vi "RT Write to Serial.vi"(4 "FPGA VI Reference in":refnum<k20>, 5 "FPGA version":string="N/A", 6 "RT Main version":string="N/A", 7 "error in":errorcluster, 8 "timeout in ms":i32=20, 9 "queue in":refnum<queue>, 10 "port name in":refnum<visa-resource-name>) -> (0 "error out":errorcluster, 2 "message dequeued?":bool, 3 "port name out":refnum<visa-resource-name>)   [LabVIEW 2018]
uses:
  Type Def Ctrls/RT ctrls/data summary.ctl
  <vilib>/Utility/error.llb/whitespace.ctl
  <vilib>/NI_Real-Time Target Support.lvlib
panel:
  out "concatenated string":string
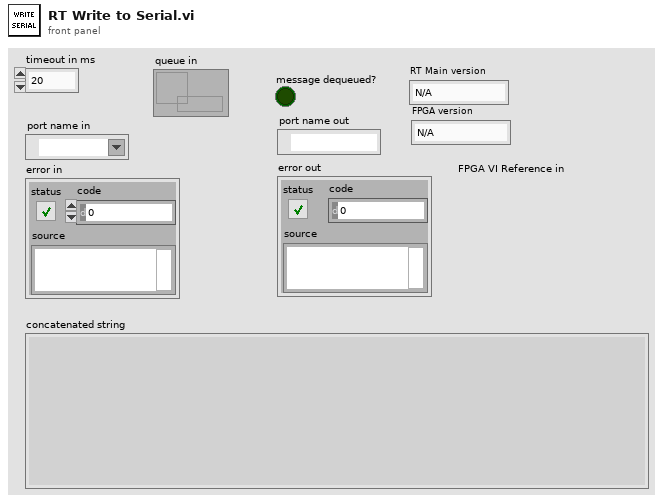
[diagram p1: front panel]
types:
  T1 = typedef "data summary.ctl" = cluster{"TIMESTAMP":dbl, "INPUT_CHN_DATA":sgl[], "OUTPUT_CHN_DATA":sgl[], "CJC_TEMPERATURE":sgl, "RELAY_SETTING":u32, "REQUEST_ID":u64, "update_system_status?":bool, "update_error_log?":bool}
  T2 = cluster{"0. connect/reconnect?":bool, "last: disconnect?":bool, "slow serial port init delay":u32}
  T3 = cluster{"2: expecting response?":bool, "expected max length":u32}
  T4 = cluster{"1: do writing?":bool, "write buffer":string}
  T5 = typedef "whitespace.ctl" = u16
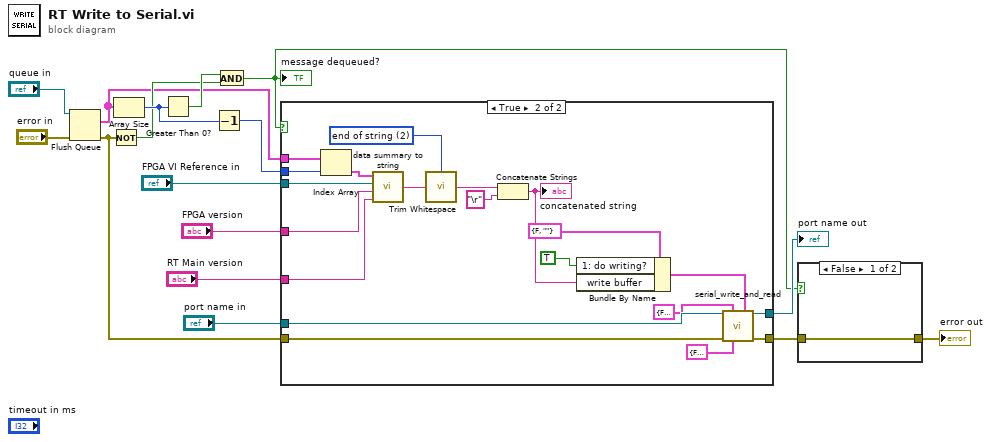
[diagram p0: block diagram]
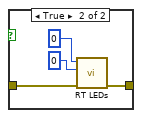
[diagram p2: hidden frame]
diagram:
  n1 = Flush Queue(queue="queue in", error in (no error)="error in") -> (remaining elements=w2:T1[], error out=w10:errorcluster)  [unwired: 1 out]
  n2 = Not(x=w10) -> (.not. x?=w7:bool)
  n3 = Array Size(array=w2) -> (size(s)=w9:i32)
  n4 = Greater Than 0?(x=w9) -> (x > 0?=w8:bool)
  n5 = Decrement(x=w9) -> (x-1=w1:i32)
  n6 = And(x=w8, y=w7) -> (x .and. y?=w6:bool)
  "message dequeued?" <- w6
  n7 = case shown="True" w6 {
    tunnel: "port name in" -> [w17 w38]
    tunnel: w10 -> [w18 w37]
    tunnel: [w18 w36] -> w14
    tunnel: [w17 w35] -> w13
    tunnel: "RT Main version" -> [_ w25]
    tunnel: "FPGA version" -> [_ w24]
    tunnel: "FPGA VI Reference in" -> [_ w23]
    tunnel: w2 -> [_ w21]
    tunnel: w1 -> [_ w20]
    frame False {
    }
    frame True {
      w34 = T5 2 items=["both", "start of string", "end of string"] ("location (both)")
      n8 = Index Array(array=w21, index=w20) -> (element=w19:T1)
      n9 = call "data summary to string.vi"("RT Main version"=w25, "FPGA version"=w24, "FPGA VI Reference in"=w23, "data summary"=w19) -> ("data summary string"=w22:string)
      n10 = call <vilib>:"Trim Whitespace.vi"("string"=w22, "location (both)"=w34) -> ("trimmed string"=w33:string)
      n11 = Concatenate Strings(w33, "\r" ("string")) -> (w29:string)
      "concatenated string" <- w29
      n12 = Bundle By Name(cluster=T4 {"1: do writing?"=FALSE, "write buffer"=""} ("1. writing setting input"), "1: do writing?"=TRUE, "write buffer"=w29) -> (w27:T4)
      n13 = call "serial_write_and_read.vi"("port name in"=w38, "0 and last: Connection/Reconnection setting"=T2 {"0. connect/reconnect?"=FALSE, "last: disconnect?"=FALSE, "slow serial port init delay"=0}, "1. writing setting input"=w27, "error in"=w37, "2. reading settings input"=T3 {"2: expecting response?"=FALSE, "expected max length"=4096}) -> ("port name out"=w35:refnum<visa-resource-name>, "error out"=w36:errorcluster)  [unwired: 8 in, 1 out]
    }
  }
  "port name out" <- w13
  n14 = case shown="False" w6 {
    tunnel: [w39 w43] -> w12
    tunnel: w14 -> [w39 w40]
    frame False {
    }
    frame True {
      n15 = call <vilib>:"RT LEDs.vi"("error in (no error)"=w40, "State"=0, "LED Num"=0) -> ("error out"=w43:errorcluster)  [unwired: 3 in, 1 out]
    }
  }
  "error out" <- w12
